vi "运维调试_总磷总氮.vi"() -> ()   [LabVIEW 2016, in "斯坦道总磷总氮.lvlib"]
uses:
  <vilib>/Utility/miscctls.llb/LVPointTypeDef.ctl
  <vilib>/Utility/config.llb/NI_LVConfig.lvlib
  <vilib>/ptbypt/NI_PtbyPt.lvlib
panel:
  in  "模块启用":bool
  in  "串口设置":bool
  in  "备用系数一键写入":bool
  in  "公式一键写入":bool
  in  "流程路径":path=path "C:/Users/std/Documents/斯坦道流程文件/流程.xml"
  in  "曲线模型":cluster{"X^2":dbl, "X":dbl, "B":dbl}(xcontrol)
  out "字符串 2":string
  in  "质控参数设置":bool
  in  "总氮自动测试量程配置":T1
  in  "总磷自动测试量程配置":T1
  out "温度2":sgl
  out "温度1":sgl
  out "ADC":sgl
  out "总氮稀释倍数":dbl
  out "固件版本号":string
  in  "数组":string[](array[string])
  in  "备用系数写入":bool
  in  "备用系数读取":bool
  in  "备用系数":T2
  in  "量程切换阈值写入":bool
  in  "量程切换阈值读取":bool
  in  "量程切换阈值":cluster{"阈值":dbl, "标液浓度":dbl}
  in  "参数下拉列表":enum16{"总磷", "总氮"}(ring)
  in  "量程下拉列表":enum16{"低量程", "高量程"}(ring)
  in  "测量模式下拉列表":enum16{"水样测量", "零点核查", "跨度核查", "标样核查", "加标回收"}(ring)
  in  "公式":cluster{"X^2":dbl, "X":dbl, "b":dbl}
  in  "写公式":bool
  in  "读公式":bool
  in  "返回":bool
  in  "设置":bool
  out "序列号":string="序列号"
  out "总氮测量数据":T3(xcontrol)
  out "总磷测量数据":T3(xcontrol)
  out "集成报警信息":string
  out "定时启动":bool
  out "总磷总氮运行状态":T4(xcontrol)
  in  "停止":bool
  in  "手动启动":bool
  in  "单步测试":bool
  in  "总磷氨氮调试":u16[](xcontrol)
  out "F3":sgl format="%#.6f"
  out "F2":sgl format="%#.6f"
  out "F1":sgl format="%#.6f"
  out "F0":sgl format="%#.6f"
  out "多列列表框":i32(listbox)
  # "参数设置"
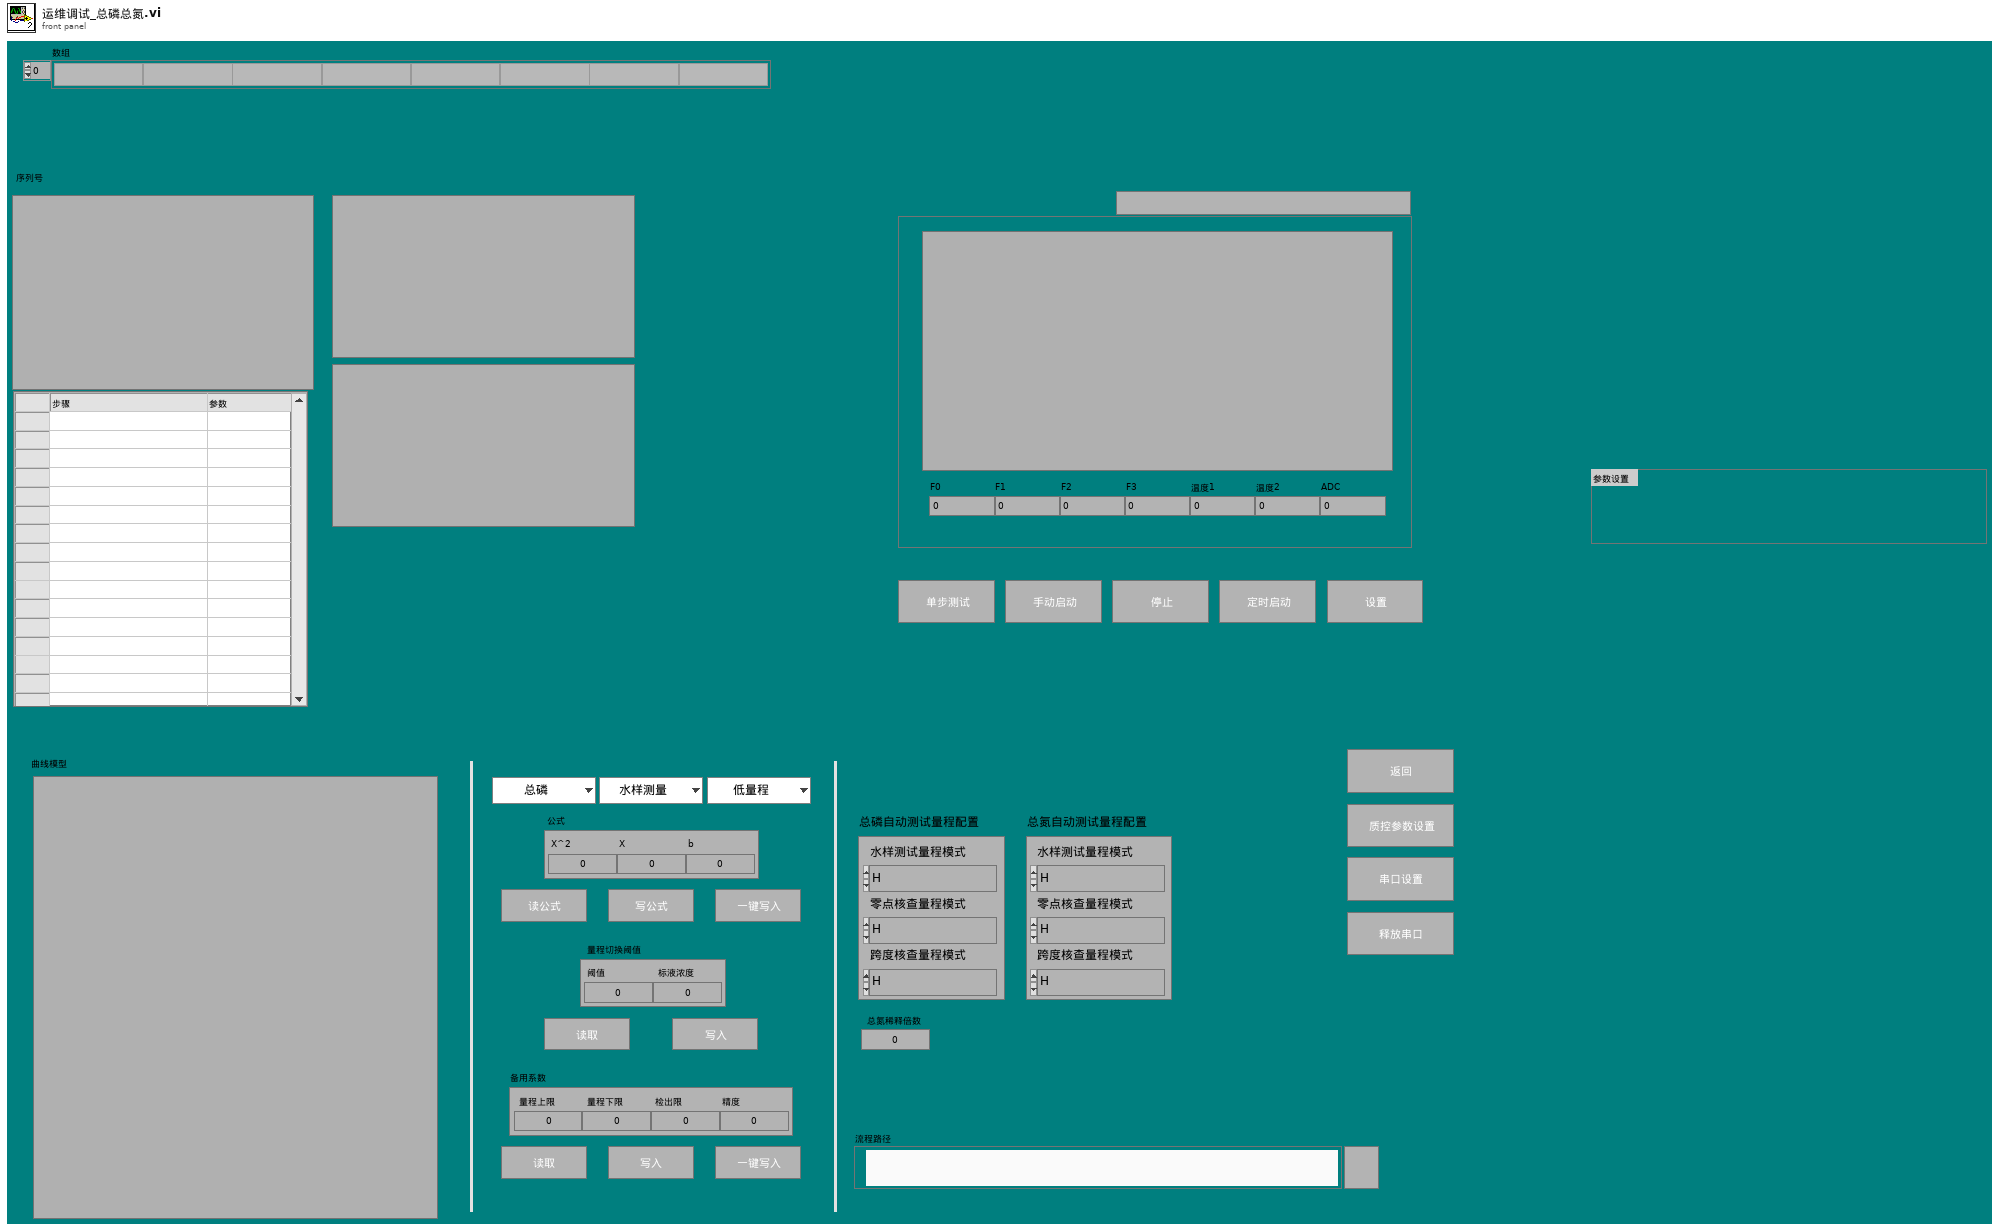
[diagram p1: front panel]
types:
  T1 = cluster{"水样测试量程模式":enum16{"H", "L", "AUTO"}, "空白核查量程模式":enum16{"H", "L", "AUTO"}, "跨度核查量程模式":enum16{"H", "L", "AUTO"}}
  T2 = cluster{"量程上限":dbl, "量程下限":dbl, "检出限":dbl, "精度":dbl}
  T3 = cluster{"flowid":u16, "测量精度":u16, "测量数据区":cluster{"因子编码":u32, "单位":u16, "标样参考值":sgl, "水样数据时间":timestamp, "水样实测值":sgl, "水样数据标识":string, "标样数据时间":timestamp, "标样实测值":sgl, "标样数据标识":string, "空白数据时间":timestamp, "空白实测值":sgl, "空白数据标识":string, "零点核查数据时间":timestamp, "零点核查实测值":sgl, "零点核查数据标识":string, "跨度核查数据时间":timestamp, "跨度核查实测值":sgl, "跨度核查数据标识":string, "加标回收数据时间":timestamp, "加标回收实测值":sgl, "加标回收数据标识":string, "平行样数据时间":timestamp, "平行样实测值":sgl, "平行样数据标识":string, "F0":sgl, "F1":sgl, "F2":sgl, "F3":sgl, "F4":sgl, "F5":sgl, "F6":sgl, "F7":sgl, "温度":sgl, "湿度":sgl, "X值":sgl}}
  T4 = cluster{"系统时间":timestamp, "工作状态":enum16{"空闲", "水样测试", "标样核查", "零点核查", "跨度核查", "空白测试", "平行样测试", "加标回收", "空白校准", "标样校准", "初始化（清洗）"}, "测量模式":enum16{"待机", "连续模式", "周期模式", "定点模式", "受控模式", "手动模式"}, "告警代码":enum16{"无告警", "缺试剂告警", "缺水样告警", "缺蒸馏水告警", "缺标液告警", "仪表漏液告警", "标定异常告警", "超量程告警", "加热异常", "低试剂预警", "超上限告警", "超下限告警", "仪表内部其他异常", "滴定异常告警", "电极异常告警", "量程切换告警", "参数设置告警", "PH电极电位异常", "电导率电极异常", "浊度光度异常", "溶解氧电极异常", "溶解氧光强异常", "温度异常告警", "PH异常告警", "溶解氧异常告警", "电导率异常告警", "浊度异常告警", "叶绿素异常告警", "藻密度异常告警", "蓝绿藻异常告警", "ORP异常告警", "氨氮异常告警", "清洁刷异常告警", "SD卡异常告警", "蓝牙异常告警", "Wifi异常告警", "流程异常告警"}, "故障代码":enum16{"无故障", "电机故障", "温度故障", "通讯故障", "滴定故障"}, "日志代码":u16, "软件版本":u16, "F0":sgl, "F1":sgl, "F2":sgl, "F3":sgl, "T":sgl, "H":sgl, "id":u16, "flowid":u16, "量程":u16, "总磷控温温度1":sgl, "营养盐控温温度2":sgl, "ADC":sgl}
  T5 = enum16{"启动测量", "标样核查", "零点核查", "跨度核查", "空白测试", "平行样测试", "加标回收", "空白校准", "标样校准", "初始化（清洗）", "停止测试", "仪器重启", "校时", "模式设置", "测量间隔设置"}
  T6 = cluster{"仪器测试类型":enum16{"启动测量", "标样核查", "零点核查", "跨度核查", "空白测试", "平行样测试", "加标回收", "空白校准", "标样校准", "初始化（清洗）", "停止测试", "仪器重启", "校时", "模式设置", "测量间隔设置"}, "周期设置类型":enum16{"定点启动", "间隔启动"}, "定时功能启用":bool, "定时间隔":dbl, "24H周期设置":bool[], "零点核查时间":u16, "跨度核查时间":u16, "质控频次":enum16{"关闭", "每天", "星期一", "星期二", "星期三", "星期四", "星期五", "星期六", "星期日"}}
  T7 = enum16{"关闭", "每天", "星期一", "星期二", "星期三", "星期四", "星期五", "星期六", "星期日"}
  T8 = enum32{"Bad", "Idle", "Run top level", "Running"}
  T9 = typedef "LVDateTimeRec.ctl" = cluster{"秒数的小数部分":dbl, "秒":i32, "分":i32, "时":i32, "日":i32, "月":i32, "年":i32, "天数（周）":i32, "天数（年）":i32, "DST":i32}
  T10 = typedef "LVPointTypeDef.ctl" = cluster{"Horizontal":i16, "Vertical":i16}
  T11 = cluster{"因子编码":u32, "单位":u16, "标样参考值":sgl, "水样数据时间":timestamp, "水样实测值":sgl, "水样数据标识":string, "标样数据时间":timestamp, "标样实测值":sgl, "标样数据标识":string, "空白数据时间":timestamp, "空白实测值":sgl, "空白数据标识":string, "零点核查数据时间":timestamp, "零点核查实测值":sgl, "零点核查数据标识":string, "跨度核查数据时间":timestamp, "跨度核查实测值":sgl, "跨度核查数据标识":string, "加标回收数据时间":timestamp, "加标回收实测值":sgl, "加标回收数据标识":string, "平行样数据时间":timestamp, "平行样实测值":sgl, "平行样数据标识":string, "F0":sgl, "F1":sgl, "F2":sgl, "F3":sgl, "F4":sgl, "F5":sgl, "F6":sgl, "F7":sgl, "温度":sgl, "湿度":sgl, "X值":sgl}
  T12 = enum16{"空闲", "水样测试", "标样核查", "零点核查", "跨度核查", "空白测试", "平行样测试", "加标回收", "空白校准", "标样校准", "初始化（清洗）"}
  T13 = typedef "NI_LVConfig.lvlib/Config Data RefNum.ctl" = refnum<k1>
  T14 = cluster{"启动模式":enum16{"跨度核查", "水样测量", "空白核查", "标样核查", "加标回收"}, "启动参数":u16, "量程":enum16{"低量程", "高量程"}}
  T15 = cluster{"时间标识":timestamp, "设备":string, "日志信息":string, "流程参数":string}
  T16 = cluster{"时间标识":timestamp, "设备":string, "日志信息":string}
  T17 = enum16{"无告警", "缺试剂告警", "缺水样告警", "缺蒸馏水告警", "缺标液告警", "仪表漏液告警", "标定异常告警", "超量程告警", "加热异常", "低试剂预警", "超上限告警", "超下限告警", "仪表内部其他异常", "滴定异常告警", "电极异常告警", "量程切换告警", "参数设置告警", "PH电极电位异常", "电导率电极异常", "浊度光度异常", "溶解氧电极异常", "溶解氧光强异常", "温度异常告警", "PH异常告警", "溶解氧异常告警", "电导率异常告警", "浊度异常告警", "叶绿素异常告警", "藻密度异常告警", "蓝绿藻异常告警", "ORP异常告警", "氨氮异常告警", "清洁刷异常告警", "SD卡异常告警", "蓝牙异常告警", "Wifi异常告警", "流程异常告警"}
  T18 = typedef "LVRowAndColumnUnsignedTypeDef.ctl" = cluster{"Row":u32, "Column":u32}
  T19 = cluster{"参数下拉列表":enum16{"总磷", "总氮"}, "测量模式下拉列表":enum16{"水样测量", "零点核查", "跨度核查", "标样核查", "加标回收"}, "量程下拉列表":enum16{"低量程", "高量程"}}
  T20 = cluster{"站号":u16, "量程切换":enum32{"H", "L", "AUTO"}, "控制命令":enum16{"启动测量", "标样核查", "零点核查", "跨度核查", "空白测试", "平行样测试", "加标回收", "空白校准", "标样校准", "初始化（清洗）", "停止测试", "仪器重启", "校时", "模式设置", "测量间隔设置"}, "模式设置":enum16{"待机", "连续模式", "周期模式", "定点模式", "受控模式", "手动模式"}, "测量间隔":u16}
  T21 = cluster{"总磷跨度值":dbl, "总磷零点标准液浓度":dbl, "总磷跨度标准液浓度":dbl, "总磷标准液标准浓度":dbl, "总氮跨度值":dbl, "总氮零点标准液浓度":dbl, "总氮跨度标准液浓度":dbl, "总氮标准液标准浓度":dbl}
  T22 = cluster{"确定":bool, "总磷跨度值":dbl, "总磷零点标准液浓度":dbl, "总磷跨度标准液浓度":dbl, "总磷标准液标准浓度":dbl, "总氮跨度值":dbl, "总氮零点标准液浓度":dbl, "总氮跨度标准液浓度":dbl, "总氮标准液标准浓度":dbl}
  T23 = cluster{"控制命令":enum16{"启动测量", "标样核查", "零点核查", "跨度核查", "空白测试", "平行样测试", "加标回收", "空白校准", "标样校准", "初始化（清洗）", "停止测试", "仪器重启", "校时", "模式设置", "测量间隔设置"}, "周期设置类型":enum16{"定点启动", "间隔启动"}, "定时功能启用":bool, "定时间隔":dbl, "24H周期设置":bool[], "空白核查时间":u16, "跨度核查时间":u16, "质控频次":enum16{"关闭", "每天", "星期一", "星期二", "星期三", "星期四", "星期五", "星期六", "星期日"}}
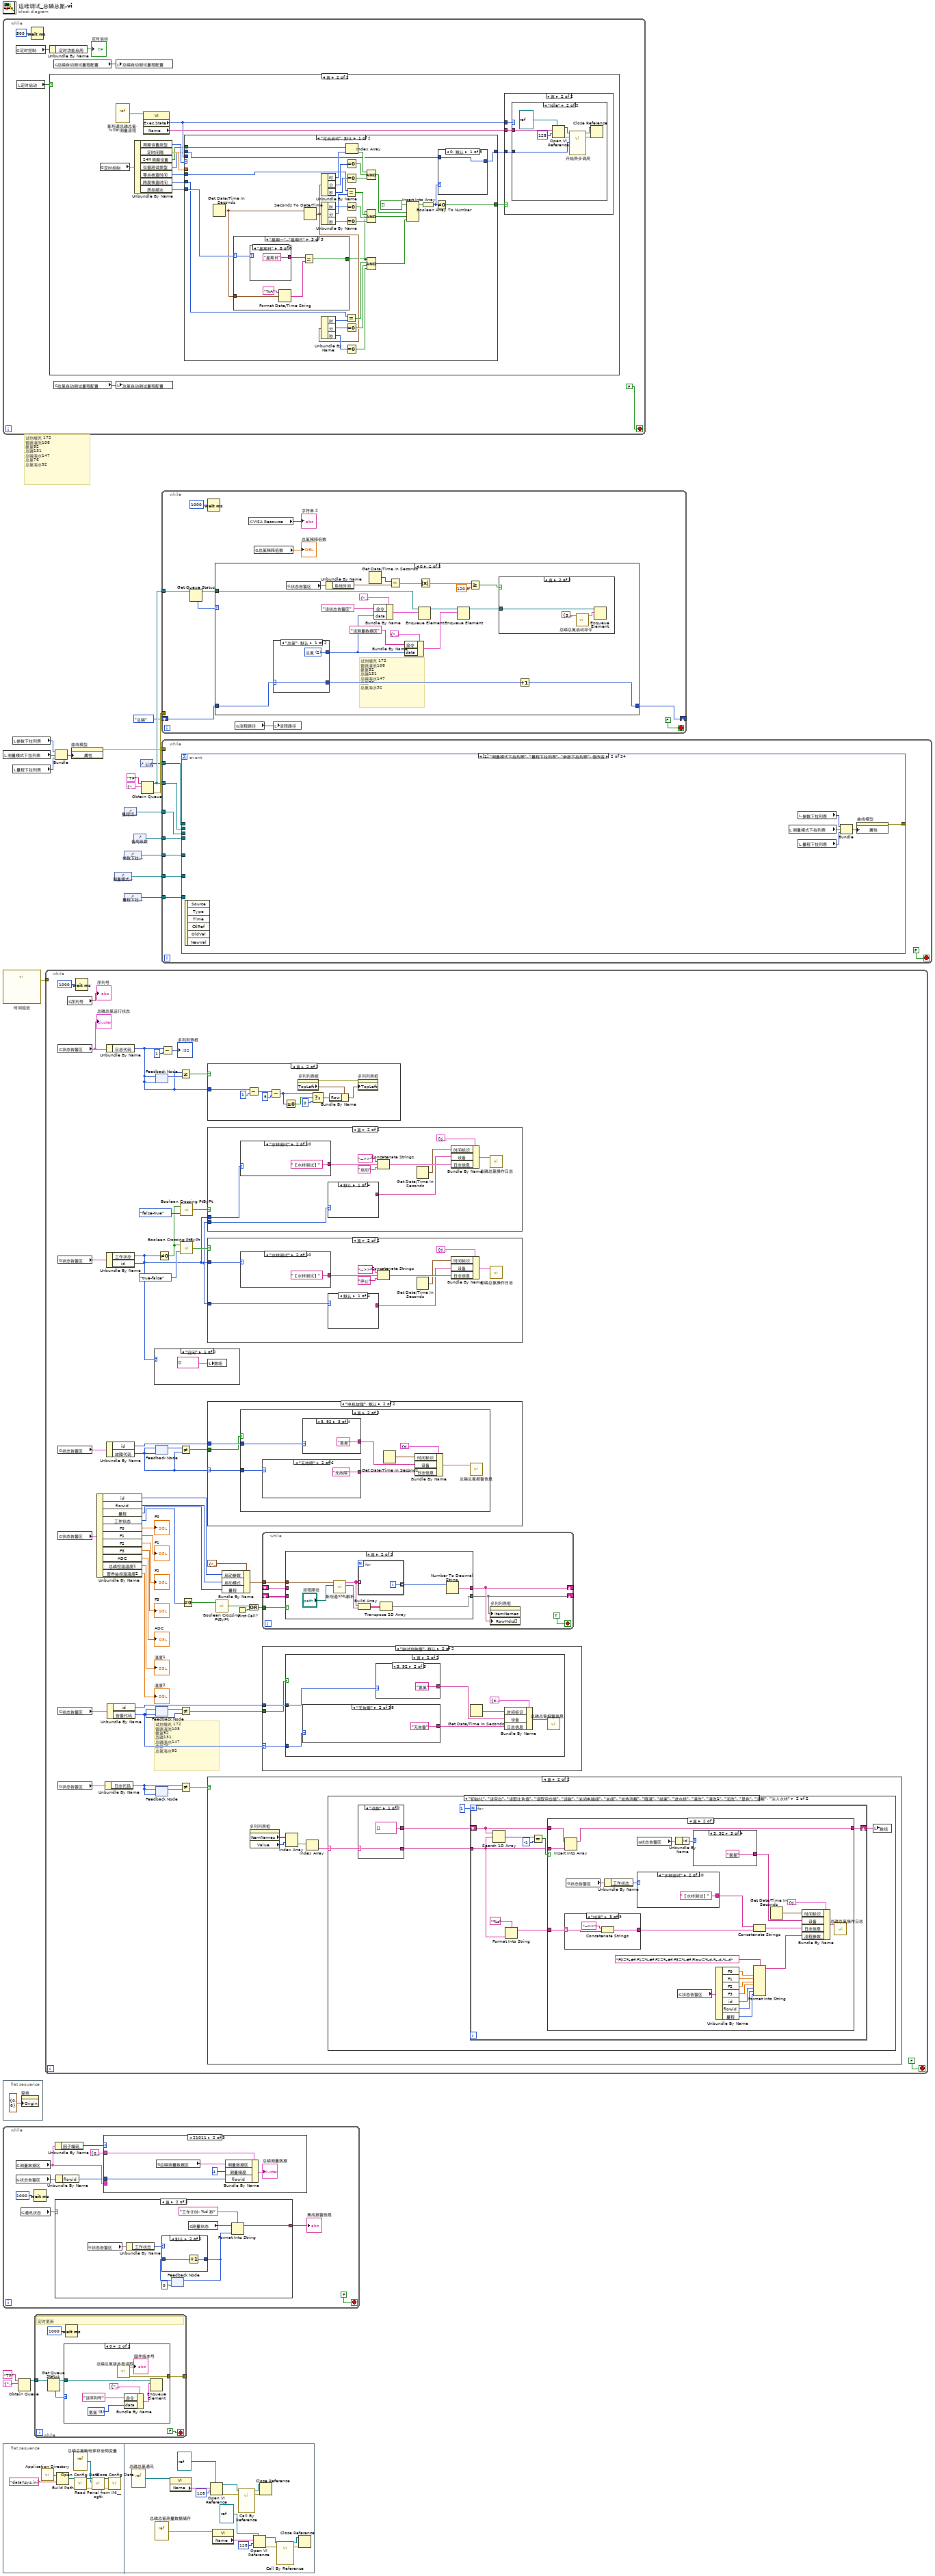
[diagram p0: block diagram]
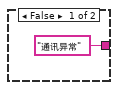
[diagram p3: hidden frame]
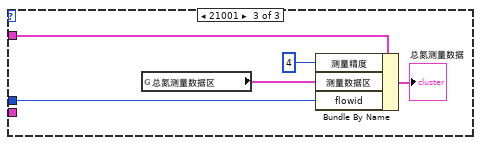
[diagram p6: hidden frame]
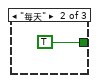
[diagram p9: hidden frame]
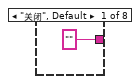
[diagram p10: hidden frame]
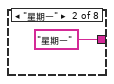
[diagram p11: hidden frame]
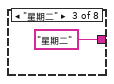
[diagram p12: hidden frame]
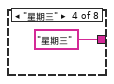
[diagram p13: hidden frame]
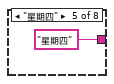
[diagram p14: hidden frame]
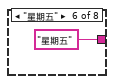
[diagram p15: hidden frame]
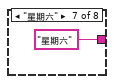
[diagram p16: hidden frame]
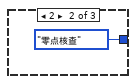
[diagram p17: hidden frame]
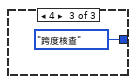
[diagram p18: hidden frame]
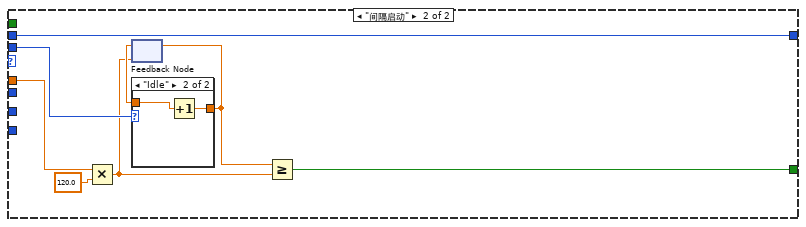
[diagram p19: hidden frame]
diagram:
  # "试剂填充 172 \n管路清洗108\n氨氮92\n总磷131\n总磷海水147\n总氮76\n总氮海水92"
  n1 = while {
    stop <- FALSE stop-if-true
    n2 = global read "总磷总氮断电保存全局变量.vi" "定时控制"() -> (w22:T6)
    n3 = local read "定时启动"() -> (w25:bool)
    n4 = Wait (ms)(milliseconds to wait=u32 500 ("等待时间（毫秒）")) -> ()  [unwired: 1 out]
    n5 = Unbundle By Name(w22) -> ("定时功能启用"=→"定时启动":bool)
    n6 = case shown="真" w25 {
      frame False {
      }
      frame True {
        n7 = global read "总磷总氮断电保存全局变量.vi" "定时控制"() -> (w40:T6)
        n8 = vi-ref "斯坦道总磷总氮.lvlib:测量流程.vi"() -> (w39:refnum<vi>)
        n9 = Unbundle By Name(w40) -> ("周期设置类型"=w37:enum16{"定点启动", "间隔启动"}, "定时间隔"=w35:dbl, "24H周期设置"=w34:bool[], "仪器测试类型"=w33:T5, "零点核查时间"=w32:u16, "跨度核查时间"=w31:u16, "质控频次"=w30:T7)
        n10 = property class="VI"(reference=w39) -> ("Exec.State"=w36:T8, "Name"=w38:string)  [unwired: 1 in, 2 out]
        n11 = case shown="\"定点启动\", 默认" w37 {
          tunnel: w35 -> [_ w97]
          tunnel: w34 -> [w65 _]
          tunnel: w36 -> [_ w100]
          tunnel: [w43 w95] -> w28
          tunnel: w33 -> [w41 w93]
          tunnel: [w69 w93] -> w29
          tunnel: w30 -> [w68 _]
          tunnel: w32 -> [w61 _]
          tunnel: w31 -> [w50 _]
          frame "定点启动", Default {
            n12 = Get Date/Time In Seconds() -> (seconds since 1Jan1904=w67:timestamp)
            n13 = case shown="\"星期一\"..\"星期日\"" w68 {
              selector: w68 -> [_ _ w79]
              tunnel: w67 -> [_ _ w80]
              tunnel: [_ TRUE w76] -> w49
              frame "关闭", Default {
              }
              frame "每天" {
              }
              frame "星期一".."星期日" {
                n14 = case shown="\"星期日\"" w79 {
                  tunnel: ["" ("时间格式字符串(%c)") "星期一" ("时间格式字符串(%c)") "星期二" ("时间格式字符串(%c)") "星期三" ("时间格式字符串(%c)") "星期四" ("时间格式字符串(%c)") "星期五" ("时间格式字符串(%c)") "星期六" ("时间格式字符串(%c)") "星期日" ("时间格式字符串(%c)")] -> w78
                  frame "关闭", Default {
                  }
                  frame "星期一" {
                  }
                  frame "星期二" {
                  }
                  frame "星期三" {
                  }
                  frame "星期四" {
                  }
                  frame "星期五" {
                  }
                  frame "星期六" {
                  }
                  frame "星期日" {
                  }
                }
                n15 = Format Date/Time String(time format string (%c)="%A" ("时间格式字符串(%c)"), seconds (now)=w80) -> (date/time string=w77:string)  [unwired: 1 in]
                n16 = Equal?(x=w78, y=w77) -> (x = y?=w76:bool)
              }
            }
            n17 = Seconds To Date/Time(time stamp (now)=w67) -> (date time rec=w51:T9)  [unwired: 1 in]
            n18 = Unbundle By Name(w51) -> ("时"=w74:i32, "分"=w72:i32, "秒"=w73:i32)
            n19 = Unbundle By Name(w51) -> ("时"=w62:i32, "分"=w64:i32, "秒"=w63:i32)
            n20 = Unbundle By Name(w51) -> ("时"=w54:i32, "分"=w52:i32, "秒"=w53:i32)
            n21 = Equal?(x=w61, y=w62) -> (x = y?=w60:bool)
            n22 = Equal?(x=w50, y=w54) -> (x = y?=w55:bool)
            n23 = Equal To 0?(x=w72) -> (x = 0?=w71:bool)
            n24 = Equal To 0?(x=w73) -> (x = 0?=w70:bool)
            n25 = Equal To 0?(x=w64) -> (x = 0?=w59:bool)
            n26 = Equal To 0?(x=w63) -> (x = 0?=w58:bool)
            n27 = Equal To 0?(x=w52) -> (x = 0?=w56:bool)
            n28 = Equal To 0?(x=w53) -> (x = 0?=w57:bool)
            n29 = Index Array(array=w65, index=w74) -> (element=w66:bool)
            n30 = Compound Arithmetic op=AND ("复合运算")(w66, w71, w70) -> (w47:bool)
            n31 = Compound Arithmetic op=AND ("复合运算")(w49, w60, w59, w58) -> (w46:bool)
            n32 = Compound Arithmetic op=AND ("复合运算")(w49, w55, w56, w57) -> (w45:bool)
            n33 = Insert Into Array(array=bool[] [], new element #1=w47, new element #2=w46, new element #3=w45) -> (w44:bool[])  [unwired: 1 in]
            n34 = Boolean Array To Number(Boolean array=w44) -> (number=w42:u32)
            n35 = Not Equal To 0?(x=w42) -> (x != 0?=w43:bool)
            n36 = case shown="0, 默认" w42 {
              tunnel: [w90 T5."零点核查" ("控制命令") T5."跨度核查" ("控制命令")] -> w69
              tunnel: w41 -> [w90 _ _]
              frame 0, Default {
              }
              frame 2 {
              }
              frame 4 {
              }
            }
          }
          frame "间隔启动" {
            n37 = Multiply(x=w97, y=120.0) -> (x*y=w94:dbl)
            n38 = feedback #1(w94) -> (w99:dbl)
            n39 = case shown="\"Idle\"" w100 {
              tunnel: w99 -> [_ w102]
              tunnel: [_ w101] -> w98
              frame "Bad", Default {
              }
              frame "Idle" {
                n40 = Increment(x=w102) -> (x+1=w101:dbl)
              }
            }
            n41 = feedback-in #1(w98) -> ()
            n42 = Greater Or Equal?(x=w98, y=w94) -> (x >= y?=w95:bool)
          }
        }
        n43 = case shown="真" w28 {
          tunnel: w38 -> [_ w105]
          tunnel: w29 -> [_ w104]
          tunnel: w36 -> [_ w103]
          frame False {
          }
          frame True {
            n44 = case shown="\"Idle\"" w103 {
              tunnel: w105 -> [_ w109]
              tunnel: w104 -> [_ w106]
              frame "Bad", Default {
              }
              frame "Idle" {
                n45 = Open VI Reference(type specifier VI Refnum (for type only)=refnum<vi> refnum, vi path=w109, options=128 ("选项")) -> (vi reference=w110:refnum<vi>, error out=w111:errorcluster)  [unwired: 3 in]
                n46 = call-by-ref "开始异步调用"(reference=w110, error in=w111, "控制命令"=w106) -> (reference out=w112:refnum<vi>, error out=w113:errorcluster)  [unwired: 11 in]
                n47 = Close Reference(reference=w112, error in (no error)=w113) -> ()  [unwired: 1 out]
              }
            }
          }
        }
      }
    }
    n48 = global read "总磷总氮断电保存全局变量.vi" "总磷自动测试量程配置"() -> (w23:T1)
    n49 = global read "总磷总氮断电保存全局变量.vi" "总氮自动测试量程配置"() -> (w24:T1)
    n50 = local write "总磷自动测试量程配置"(w23) -> ()
    n51 = local write "总氮自动测试量程配置"(w24) -> ()
  }
  n52 = local read "测量模式下拉列表"() -> (w3:enum16{"水样测量", "零点核查", "跨度核查", "标样核查", "加标回收"})
  n53 = call "时间延迟"() -> ("error out"=w9:errorcluster)  [unwired: 11 in]
  n54 = flat-sequence {
    frame #0 {
      n55 = property on="窗格" class="Pane"("Origin"=T10 {"Horizontal"=0, "Vertical"=0} ("原点")) -> ()  [unwired: 2 in, 2 out]
    }
  }
  n56 = while {
    stop <- FALSE stop-if-true
    n57 = global read "VAR总磷总氮全局变量.vi" "测量数据区"() -> (w121:T11)
    n58 = global read "VAR总磷总氮全局变量.vi" "状态告警区"() -> (w117:T4)
    n59 = global read "VAR总磷总氮全局变量.vi" "通讯状态"() -> (w119:bool)
    n60 = Wait (ms)(milliseconds to wait=u32 1000 ("等待时间（毫秒）")) -> ()  [unwired: 1 out]
    n61 = Unbundle By Name(w121) -> ("因子编码"=w120:u32)
    n62 = case shown="真" w119 {
      tunnel: ["通讯异常" ("集成报警信息") w126] -> w118
      frame False {
      }
      frame True {
        n63 = global read "VAR总磷总氮全局变量.vi" "状态告警区"() -> (w132:T4)
        n64 = Unbundle By Name(w132) -> ("工作状态"=w131:T12)
        n65 = feedback #2(0) -> (w129:i32)
        n66 = case shown="默认" w131 {
          tunnel: w129 -> [_ w134]
          tunnel: [_ w133] -> w127
          frame "空闲" {
          }
          frame Default {
            n67 = Increment(x=w134) -> (x+1=w133:i32)
          }
        }
        n68 = feedback-in #2(w127) -> ()
        n69 = global read "VAR总磷总氮全局变量.vi" "测量状态"() -> (w125:string)
        n70 = Format Into String(format string="工作计时: %d 秒" ("格式字符串"), initial string=w125, w127) -> (resulting string=w126:string)  [unwired: 1 in, 1 out]
      }
    }
    "集成报警信息" <- w118
    n71 = Unbundle By Name(w117) -> ("flowid"=w116:u16)
    n72 = case shown="21011" w120 {
      tunnel: w121 -> [_ _ _]
      tunnel: w116 -> [_ w137 w143]
      tunnel: T3 {"flowid"=0, "测量精度"=0, "测量数据区"={"因子编码"=0, "单位"=0, "标样参考值"=0.0, "水样数据时间"=timestamp(0 s since 1904-01-01), "水样实测值"=0.0, "水样数据标识"="", "标样数据时间"=timestamp(0 s since 1904-01-01), "标样实测值"=0.0, "标样数据标识"="", "空白数据时间"=timestamp(0 s since 1904-01-01), "空白实测值"=0.0, "空白数据标识"="", "零点核查数据时间"=timestamp(0 s since 1904-01-01), "零点核查实测值"=0.0, "零点核查数据标识"="", "跨度核查数据时间"=timestamp(0 s since 1904-01-01), "跨度核查实测值"=0.0, "跨度核查数据标识"="", "加标回收数据时间"=timestamp(0 s since 1904-01-01), "加标回收实测值"=0.0, "加标回收数据标识"="", "平行样数据时间"=timestamp(0 s since 1904-01-01), "平行样实测值"=0.0, "平行样数据标识"="", "F0"=0.0, "F1"=0.0, "F2"=0.0, "F3"=0.0, "F4"=0.0, "F5"=0.0, "F6"=0.0, "F7"=0.0, "温度"=0.0, "湿度"=0.0, "X值"=0.0}} ("总氮测量数据") -> [_ w136 w142]
      frame Default {
      }
      frame 21011 {
        n73 = global read "VAR总磷总氮全局变量.vi" "总磷测量数据区"() -> (w135:T11)
        n74 = Bundle By Name(cluster=w136, "测量数据区"=w135, "测量精度"=u16 4, "flowid"=w137) -> (→"总磷测量数据":T3)
      }
      frame 21001 {
        n75 = global read "VAR总磷总氮全局变量.vi" "总氮测量数据区"() -> (w140:T11)
        n76 = Bundle By Name(cluster=w142, "测量精度"=u16 4, "测量数据区"=w140, "flowid"=w143) -> (→"总氮测量数据":T3)
      }
    }
  }
  n77 = flat-sequence {
    frame #0 {
      n78 = call <vilib>:"Application Directory.vi"() -> ("Application Directory"=w152:path)
      n79 = Build Path(base path=w152, name or relative path="data\\sys.ini" ("名称或相对路径")) -> (appended path=w150:path)
      n80 = vi-ref "总磷总氮断电保存全局变量.vi"() -> (w148:refnum<vi>)
      n81 = call <vilib>:"Open Config Data.vi"("configuration file path"=w150) -> ("error out"=w146:errorcluster, "refnum"=w149:T13)  [unwired: 8 in, 1 out]
      n82 = call <userlib>:"Read Panel from INI__ogtk.vi"("error in (no error)"=w146, "VI ref"=w148, "refnum"=w149) -> ("error out"=w145:errorcluster, "refnum out"=w147:T13)  [unwired: 7 in]
      n83 = call <vilib>:"Close Config Data.vi"("error in (no error)"=w145, "refnum"=w147) -> ()  [unwired: 8 in, 2 out]
    }
    frame #1 {
      n84 = vi-ref "总磷总氮通讯.vi"() -> (w168:refnum<vi>)
      n85 = vi-ref "总磷总氮测量数据储存.vi"() -> (w160:refnum<vi>)
      n86 = property class="VI"(reference=w168) -> ("Name"=w167:string)  [unwired: 1 in, 2 out]
      n87 = Open VI Reference(type specifier VI Refnum (for type only)=refnum<vi> refnum, vi path=w167, options=128 ("选项")) -> (vi reference=w165:refnum<vi>, error out=w163:errorcluster)  [unwired: 3 in]
      n88 = property class="VI"(reference=w160) -> ("Name"=w153:string)  [unwired: 1 in, 2 out]
      n89 = call-by-ref "?"(reference=w165, error in=w163) -> (reference out=w161:refnum<vi>, error out=w162:errorcluster)  [unwired: 12 in]
      n90 = Open VI Reference(type specifier VI Refnum (for type only)=refnum<vi> refnum, vi path=w153, options=128 ("选项")) -> (vi reference=w155:refnum<vi>, error out=w157:errorcluster)  [unwired: 3 in]
      n91 = Close Reference(reference=w161, error in (no error)=w162) -> ()  [unwired: 1 out]
      n92 = call-by-ref "?"(reference=w155, error in=w157) -> (reference out=w159:refnum<vi>, error out=w158:errorcluster)  [unwired: 12 in]
      n93 = Close Reference(reference=w159, error in (no error)=w158) -> ()  [unwired: 1 out]
    }
  }
  n94 = local read "参数下拉列表"() -> (w2:enum16{"总磷", "总氮"})
  n95 = local read "量程下拉列表"() -> (w1:enum16{"低量程", "高量程"})
  n96 = Obtain Queue(name (unnamed)="TP" ("名称（未命名）"), element data type=cluster{"命令":string, "data":variant} {"命令"="", "data"=variant}) -> (queue out=w6:refnum<queue>)  [unwired: 3 in, 2 out]
  n97 = while {
    tunnel: w6 -> [w173]
    tunnel: [w171] -> _
    stop <- FALSE stop-if-true
    # "定时更新"
    n98 = Get Queue Status(queue=w173) -> (queue out=w170:refnum<queue>, # elements in queue=w169:i32)  [unwired: 2 in, 6 out]
    n99 = case shown="0" w169 {
      tunnel: w170 -> [_ w178]
      tunnel: [_ w175] -> w171
      frame Default {
      }
      frame 0 {
        w179 = u16 3 items=["总磷"=1, "氨氮"=3] ("站号")
        n100 = call "总磷总氮版本号读取.vi"() -> ("error out"=w175:errorcluster, "固件版本号"=→"固件版本号":string)  [unwired: 10 in]
        n101 = Bundle By Name(cluster=cluster{"命令":string, "data":variant} {"命令"="", "data"=variant} ("元素"), "命令"="读序列号", "data"=w179) -> (w177:cluster{"命令":string, "data":variant})
        n102 = Enqueue Element(queue=w178, element=w177) -> ()  [unwired: 2 in, 3 out]
      }
    }
    n103 = Wait (ms)(milliseconds to wait=u32 1000 ("等待时间（毫秒）")) -> ()  [unwired: 1 out]
  }
  n104 = while {
    tunnel: w9 -> [_]
    stop <- FALSE stop-if-true
    # "试剂填充 172 \n管路清洗108\n氨氮92\n总磷131\n总磷海水147\n总氮76\n总氮海水92"
    n105 = global read "VAR总磷总氮全局变量.vi" "状态告警区"() -> (w215:T4)
    "总磷总氮运行状态" <- w215
    n106 = global read "VAR总磷总氮全局变量.vi" "状态告警区"() -> (w202:T4)
    n107 = global read "VAR总磷总氮全局变量.vi" "状态告警区"() -> (w207:T4)
    n108 = global read "VAR总磷总氮全局变量.vi" "状态告警区"() -> (w223:T4)
    n109 = global read "VAR总磷总氮全局变量.vi" "状态告警区"() -> (w212:T4)
    n110 = global read "VAR总磷总氮全局变量.vi" "状态告警区"() -> (w200:T4)
    n111 = global read "VAR总磷总氮全局变量.vi" "序列号"() -> (→"序列号":string)
    n112 = Wait (ms)(milliseconds to wait=u32 1000 ("等待时间（毫秒）")) -> ()  [unwired: 1 out]
    n113 = Unbundle By Name(w223) -> ("id"=w220:u16, "flowid"=w222:u16, "量程"=w221:u16, "工作状态"=w190:T12, "F0"=→"F0":sgl, "F1"=→"F1":sgl, "F2"=→"F2":sgl, "F3"=→"F3":sgl, "ADC"=→"ADC":sgl, "总磷控温温度1"=→"温度1":sgl, "营养盐控温温度2"=→"温度2":sgl)
    n114 = Unbundle By Name(w200) -> ("日志代码"=w199:u16)
    n115 = Unbundle By Name(w215) -> ("日志代码"=w196:u16)
    n116 = Unbundle By Name(w202) -> ("工作状态"=w183:T12, "id"=w182:u16)
    n117 = Unbundle By Name(w207) -> ("id"=w206:u16, "故障代码"=w203:enum16{"无故障", "电机故障", "温度故障", "通讯故障", "滴定故障"})
    n118 = Unbundle By Name(w212) -> ("id"=w211:u16, "告警代码"=w208:T17)
    n119 = case shown="\"空闲\"" w183 {
      frame "空闲" {
        n120 = local write "数组"(string[] [] ("数组")) -> ()
      }
      frame "水样测试", Default {
      }
    }
    n121 = feedback-in #3(w196) -> ()
    n122 = feedback #3(w196) -> (w228:u16)
    n123 = feedback #4(w203) -> (w204:enum16{"无故障", "电机故障", "温度故障", "通讯故障", "滴定故障"})
    n124 = feedback-in #4(w203) -> ()
    n125 = feedback #5(w208) -> (w209:T17)
    n126 = feedback-in #5(w208) -> ()
    n127 = feedback #6(w199) -> (w201:u16)
    n128 = feedback-in #6(w199) -> ()
    n129 = Not Equal To 0?(x=w183) -> (x != 0?=w185:bool)
    n130 = Subtract(x=w196, y=1) -> (x-y=→"多列列表框":i32)
    n131 = Not Equal?(x=w196, y=w228) -> (x != y?=w227:bool)
    n132 = Not Equal?(x=w204, y=w203) -> (x != y?=w205:bool)
    n133 = Not Equal?(x=w209, y=w208) -> (x != y?=w210:bool)
    n134 = Not Equal?(x=w199, y=w201) -> (x != y?=w198:bool)
    n135 = call <vilib>:"Boolean Crossing PtByPt.vi"("direction"=enum16{"either", "false-true", "true-false"}."false-true", "input"=w185) -> ("crossing"=w187:bool)  [unwired: 1 in]
    n136 = call <vilib>:"Boolean Crossing PtByPt.vi"("direction"=enum16{"either", "false-true", "true-false"}."true-false", "input"=w185) -> ("crossing"=w184:bool)  [unwired: 1 in]
    n137 = Not Equal To 0?(x=w190) -> (x != 0?=w225:bool)
    n138 = case shown="真" w227 {
      tunnel: w196 -> [_ w438]
      frame False {
      }
      frame True {
        n139 = Subtract(x=w438, y=1) -> (x-y=w436:i32)
        n140 = Subtract(x=w436, y=5) -> (x-y=w440:i32)
        n141 = Greater Or Equal To 0?(x=w440) -> (x >= 0?=w439:bool)
        n142 = property on="多列列表框" class="MCListbox (严格)"() -> (error out=w444:errorcluster, "TopLeft"=w445:T18)  [unwired: 2 in, 1 out]
        n143 = Select(t=w440, s=w439, f=0) -> (s? t:f=w441:i32)
        n144 = Bundle By Name(cluster=w445, "Row"=w441) -> (w446:T18)
        n145 = property on="多列列表框" class="MCListbox (严格)"(error in=w444, "TopLeft"=w446) -> ()  [unwired: 1 in, 2 out]
      }
    }
    n146 = case shown="真" w187 {
      tunnel: w183 -> [_ w255]
      tunnel: w182 -> [_ w254]
      frame False {
      }
      frame True {
        n147 = case shown="\"水样测试\"" w255 {
          tunnel: [_ "【水样测试】" ("字符串") "【标样核查】" ("字符串") "【零点核查】" ("字符串") "【跨度核查】" ("字符串") "【空白测试】" ("字符串") "【平行样测试】" ("字符串") "【加标回收】" ("字符串") "【空白校准】" ("字符串") "【标样校准】" ("字符串")] -> w262
          frame "空闲", Default {
          }
          frame "水样测试" {
          }
          frame "标样核查" {
          }
          frame "零点核查" {
          }
          frame "跨度核查" {
          }
          frame "空白测试" {
          }
          frame "平行样测试" {
          }
          frame "加标回收" {
          }
          frame "空白校准" {
          }
          frame "标样校准" {
          }
        }
        n148 = case shown="默认" w254 {
          tunnel: [_ "总磷" ("table输入") "氨氮" ("table输入") "总氮" ("table输入")] -> w258
          frame Default {
          }
          frame 1, 131 {
          }
          frame 3, 92 {
          }
          frame 2, 76 {
          }
        }
        n149 = Concatenate Strings("-->>" ("字符串"), w262, "启动" ("字符串")) -> (w261:string)
        n150 = Get Date/Time In Seconds() -> (seconds since 1Jan1904=w259:timestamp)
        n151 = Bundle By Name(cluster=T15 {"时间标识"=timestamp(0 s since 1904-01-01), "设备"="", "日志信息"="", "流程参数"=""} ("data in"), "时间标识"=w259, "设备"=w258, "日志信息"=w261) -> (w253:T15)
        n152 = call "总磷总氮操作日志.vi"("data in"=w253) -> ()  [unwired: 11 in]
      }
    }
    n153 = case shown="真" w184 {
      tunnel: w183 -> [_ w233]
      tunnel: w182 -> [_ w232]
      frame False {
      }
      frame True {
        n154 = case shown="\"水样测试\"" w233 {
          tunnel: [_ "【水样测试】" ("字符串") "【标样核查】" ("字符串") "【零点核查】" ("字符串") "【跨度核查】" ("字符串") "【空白测试】" ("字符串") "【平行样测试】" ("字符串") "【加标回收】" ("字符串") "【空白校准】" ("字符串") "【标样校准】" ("字符串")] -> w240
          frame "空闲", Default {
          }
          frame "水样测试" {
          }
          frame "标样核查" {
          }
          frame "零点核查" {
          }
          frame "跨度核查" {
          }
          frame "空白测试" {
          }
          frame "平行样测试" {
          }
          frame "加标回收" {
          }
          frame "空白校准" {
          }
          frame "标样校准" {
          }
        }
        n155 = case shown="默认" w232 {
          tunnel: [_ "总磷" ("table输入") "氨氮" ("table输入") "总氮" ("table输入")] -> w236
          frame Default {
          }
          frame 1, 131 {
          }
          frame 3, 92 {
          }
          frame 2, 76 {
          }
        }
        n156 = Concatenate Strings("-->>" ("字符串"), w240, "停止" ("字符串")) -> (w239:string)
        n157 = Get Date/Time In Seconds() -> (seconds since 1Jan1904=w237:timestamp)
        n158 = Bundle By Name(cluster=T15 {"时间标识"=timestamp(0 s since 1904-01-01), "设备"="", "日志信息"="", "流程参数"=""} ("data in"), "时间标识"=w237, "设备"=w236, "日志信息"=w239) -> (w231:T15)
        n159 = call "总磷总氮操作日志.vi"("data in"=w231) -> ()  [unwired: 11 in]
      }
    }
    n160 = case shown="\"电机故障\", 默认" w203 {
      selector: w203 -> [_ w343]
      tunnel: w206 -> [_ w344]
      tunnel: w205 -> [_ w342]
      frame "无故障" {
      }
      frame "电机故障", Default {
        n161 = case shown="真" w342 {
          tunnel: w344 -> [_ w351]
          tunnel: w343 -> [_ w346]
          frame False {
          }
          frame True {
            n162 = case shown="\"无故障\"" w346 {
              selector: w346 -> [w353 _ _ _ _ _]
              tunnel: [w352 "无故障" "电机故障" "温度故障" "通讯故障" "滴定故障"] -> w345
              frame Default {
                n163 = Format Into String(format string="%d" ("格式字符串"), initial string="未知" ("工作状态"), w353) -> (resulting string=w352:string)  [unwired: 1 in, 1 out]
              }
              frame "无故障" {
              }
              frame "电机故障" {
              }
              frame "温度故障" {
              }
              frame "通讯故障" {
              }
              frame "滴定故障" {
              }
            }
            n164 = case shown="3, 92" w351 {
              tunnel: [_ "总磷" ("table输入") "氨氮" ("table输入") "总氮" ("table输入")] -> w347
              frame Default {
              }
              frame 1, 131 {
              }
              frame 3, 92 {
              }
              frame 2, 76 {
              }
            }
            n165 = Get Date/Time In Seconds() -> (seconds since 1Jan1904=w348:timestamp)
            n166 = Bundle By Name(cluster=T16 {"时间标识"=timestamp(0 s since 1904-01-01), "设备"="", "日志信息"=""} ("data in"), "时间标识"=w348, "设备"=w347, "日志信息"=w345) -> (w349:T16)
            n167 = call "总磷总氮报警信息.vi"("data in"=w349) -> ()  [unwired: 10 in, 1 out]
          }
        }
      }
    }
    n168 = case shown="真" w198 {
      frame False {
      }
      frame True {
        n169 = property on="多列列表框" class="MCListbox (严格)"() -> ("ItemNames"=w278:string[][], "Value"=w279:i32)  [unwired: 2 in, 2 out]
        n170 = Index Array(array=w278, index (row)=w279) -> (element=w277:string[])  [unwired: 1 in]
        n171 = Index Array(array=w277) -> (element=w276:string)  [unwired: 1 in]
        n172 = case shown="\"初始化\", \"读空白\", \"读取比色值\", \"读取空白值\", \"读数\", \"关闭电磁阀\", \"关阀\", \"加热消解\", \"降温\", \"结束\", \"进水样\", \"清洗\", \"清洗1\", \"润洗\", \"显色\", \"消解\", \"注入水样\"" w276 {
          selector: w276 -> [_ w282]
          frame Default {
          }
          frame "初始化", "读空白", "读取比色值", "读取空白值", "读数", "关闭电磁阀", "关阀", "加热消解", "降温", "结束", "进水样", "清洗", "清洗1", "润洗", "显色", "消解", "注入水样" {
            n173 = case shown="\"读数\"" w282 {
              selector: w282 -> [w286 w288]
              tunnel: [w286 w288] -> w281
              tunnel: [string[] [] ("数组") "数组"] -> w280
              frame "读数" {
              }
              frame Default {
              }
            }
            n174 = for {
              N: 1 -> [_]
              tunnel: w281 -> [w290]
              shift-right: [w289] -> w283
              shift-left: w280 -> [w291]
              n175 = Search 1D Array(1D array=w291, element=w290) -> (index of element=w294:i32)  [unwired: 1 in]
              n176 = Format Into String(format string="%s" ("格式字符串"), w290) -> (resulting string=w295:string)  [unwired: 2 in, 1 out]
              n177 = Equal?(x=w294, y=-1) -> (x = y?=w292:bool)
              n178 = case shown="真" w292 {
                tunnel: w295 -> [_ w303]
                tunnel: w291 -> [w297 w307]
                tunnel: w290 -> [_ w306]
                tunnel: [w297 w305] -> w289
                frame False {
                }
                frame True {
                  n179 = Insert Into Array(array=w307, new element=w306) -> (w305:string[])  [unwired: 1 in]
                  n180 = case shown="\"结束\"" w303 {
                    selector: w303 -> [w332 w335 w338]
                    tunnel: [w332 w334 w337] -> w302
                    frame Default {
                    }
                    frame "初始化" {
                      n181 = Concatenate Strings("-->>" ("字符串"), w335) -> (w334:string)
                    }
                    frame "结束" {
                      n182 = Concatenate Strings("-->>" ("字符串"), w338) -> (w337:string)
                    }
                  }
                  n183 = global read "VAR总磷总氮全局变量.vi" "状态告警区"() -> (w301:T4)
                  n184 = Unbundle By Name(w301) -> ("工作状态"=w300:T12)
                  n185 = global read "VAR总磷总氮全局变量.vi" "状态告警区"() -> (w322:T4)
                  n186 = case shown="\"水样测试\"" w300 {
                    tunnel: [_ "【水样测试】" ("字符串") "【标样核查】" ("字符串") "【零点核查】" ("字符串") "【跨度核查】" ("字符串") "【空白测试】" ("字符串") "【平行样测试】" ("字符串") "【加标回收】" ("字符串") "【空白校准】" ("字符串") "【标样校准】" ("字符串")] -> w298
                    frame "空闲", Default {
                    }
                    frame "水样测试" {
                    }
                    frame "标样核查" {
                    }
                    frame "零点核查" {
                    }
                    frame "跨度核查" {
                    }
                    frame "空白测试" {
                    }
                    frame "平行样测试" {
                    }
                    frame "加标回收" {
                    }
                    frame "空白校准" {
                    }
                    frame "标样校准" {
                    }
                  }
                  n187 = Unbundle By Name(w322) -> ("id"=w321:u16)
                  n188 = global read "VAR总磷总氮全局变量.vi" "状态告警区"() -> (w317:T4)
                  n189 = case shown="3, 92" w321 {
                    tunnel: [_ "总磷" ("table输入") "氨氮" ("table输入") "总氮" ("table输入")] -> w319
                    frame Default {
                    }
                    frame 1, 131 {
                    }
                    frame 3, 92 {
                    }
                    frame 2, 76 {
                    }
                  }
                  n190 = Unbundle By Name(w317) -> ("F0"=w314:sgl, "F1"=w313:sgl, "F2"=w312:sgl, "F3"=w311:sgl, "id"=w310:u16, "flowid"=w309:u16, "量程"=w308:u16)
                  n191 = Concatenate Strings(w298, w302) -> (w299:string)
                  n192 = Format Into String(format string="F0=%#f,F1=%#f,F2=%#f,F3=%#f,Flow=%d-%-d-%-d" ("格式字符串"), w314, w313, w312, w311, w310, w309, w308) -> (resulting string=w315:string)  [unwired: 2 in, 1 out]
                  n193 = Get Date/Time In Seconds() -> (seconds since 1Jan1904=w318:timestamp)
                  n194 = Bundle By Name(cluster=T15 {"时间标识"=timestamp(0 s since 1904-01-01), "设备"="", "日志信息"="", "流程参数"=""} ("data in"), "时间标识"=w318, "设备"=w319, "日志信息"=w299, "流程参数"=w315) -> (w320:T15)
                  n195 = call "总磷总氮操作日志.vi"("data in"=w320) -> ()  [unwired: 11 in]
                }
              }
            }
            n196 = local write "数组"(w283) -> ()
          }
        }
      }
    }
    n197 = call <vilib>:"Boolean Crossing PtByPt.vi"("input"=w225) -> ("crossing"=w189:bool)  [unwired: 2 in]
    n198 = Bundle By Name(cluster=T14 {"启动模式"=enum."跨度核查", "启动参数"=1, "量程"=enum."低量程"} ("参数簇"), "启动参数"=w220, "启动模式"=w222, "量程"=w221) -> (w214:T14)
    n199 = First Call?() -> (First Call?: T/F=w226:bool)
    n200 = Or(x=w189, y=w226) -> (x .or. y?=w224:bool)
    n201 = while {
      tunnel: w224 -> [w424]
      tunnel: w214 -> [w423]
      shift-right: [w418] -> _
      shift-left: _ -> [w420]
      shift-right: [w419] -> _
      shift-left: _ -> [w421]
      stop <- TRUE stop-if-true
      n202 = case shown="真" w424 {
        tunnel: [w426 w434] -> w419
        tunnel: [w425 w433] -> w418
        tunnel: w423 -> [_ w428]
        tunnel: w421 -> [w426 _]
        tunnel: w420 -> [w425 _]
        frame False {
        }
        frame True {
          n203 = call "斯坦道XML解析.vi"("添加的路径"="流程路径", "参数簇"=w428) -> ("步骤时间"=w429:string[], "步骤名"=w431:string[])  [unwired: 8 in]
          n204 = for {
            tunnel: w431 -> [_] mode=indexing
            tunnel: [w435] -> w432 mode=indexing
            i -> [w435]
          }
          n205 = Build Array(w431, w429) -> (w430:string[][])
          n206 = Transpose 2D Array(2D array=w430) -> (transposed array=w433:string[][])
          n207 = Number To Decimal String(number=w432) -> (decimal integer string=w434:string[])  [unwired: 1 in]
        }
      }
      n208 = property on="多列列表框" class="MCListbox (严格)"("ItemNames"=w418, "RowHdrs[]"=w419) -> ()  [unwired: 2 in, 2 out]
    }
    n209 = case shown="\"缺试剂告警\", 默认" w208 {
      selector: w208 -> [_ w365]
      tunnel: w211 -> [_ w366]
      tunnel: w210 -> [_ w364]
      frame "无告警" {
      }
      frame "缺试剂告警", Default {
        n210 = case shown="真" w364 {
          tunnel: w366 -> [_ w373]
          tunnel: w365 -> [_ w367]
          frame False {
          }
          frame True {
            n211 = case shown="\"无告警\"" w367 {
              selector: w367 -> [w375 _ _ _ _ _ _ _ _ _ _ _ _ _ _ _ _ _ _ _ _ _ _ _ _ _ _ _ _ _ _ _ _ _ _ _ _ _]
              tunnel: [w374 "无告警" "缺试剂告警" "缺水样告警" "缺蒸馏水告警" "缺标液告警" "仪表漏液告警" "标定异常告警" "超量程告警" "加热异常" "低试剂预警" "超上限告警" "超下限告警" "仪表内部其他异常" "滴定异常告警" "电极异常告警" "量程切换告警" "参数设置告警" "PH电极电位异常" "电导率电极异常" "浊度光度异常" "溶解氧电极异常" "溶解氧光强异常" "温度异常告警" "PH异常告警" "溶解氧异常告警" "电导率异常告警" "浊度异常告警" "叶绿素异常告警" "藻密度异常告警" "蓝绿藻异常告警" "ORP异常告警" "氨氮异常告警" "清洁刷异常告警" "SD卡异常告警" "蓝牙异常告警" "WiFi异常告警" "流程异常告警"] -> w368
              frame Default {
                n212 = Format Into String(format string="%d" ("格式字符串"), initial string="未知" ("工作状态"), w375) -> (resulting string=w374:string)  [unwired: 1 in, 1 out]
              }
              frame "无告警" {
              }
              frame "缺试剂告警" {
              }
              frame "缺水样告警" {
              }
              frame "缺蒸馏水告警" {
              }
              frame "缺标液告警" {
              }
              frame "仪表漏液告警" {
              }
              frame "标定异常告警" {
              }
              frame "超量程告警" {
              }
              frame "加热异常" {
              }
              frame "低试剂预警" {
              }
              frame "超上限告警" {
              }
              frame "超下限告警" {
              }
              frame "仪表内部其他异常" {
              }
              frame "滴定异常告警" {
              }
              frame "电极异常告警" {
              }
              frame "量程切换告警" {
              }
              frame "参数设置告警" {
              }
              frame "PH电极电位异常" {
              }
              frame "电导率电极异常" {
              }
              frame "浊度光度异常" {
              }
              frame "溶解氧电极异常" {
              }
              frame "溶解氧光强异常" {
              }
              frame "温度异常告警" {
              }
              frame "PH异常告警" {
              }
              frame "溶解氧异常告警" {
              }
              frame "电导率异常告警" {
              }
              frame "浊度异常告警" {
              }
              frame "叶绿素异常告警" {
              }
              frame "藻密度异常告警" {
              }
              frame "蓝绿藻异常告警" {
              }
              frame "ORP异常告警" {
              }
              frame "氨氮异常告警" {
              }
              frame "清洁刷异常告警" {
              }
              frame "SD卡异常告警" {
              }
              frame "蓝牙异常告警" {
              }
              frame "Wifi异常告警" {
              }
              frame "流程异常告警" {
              }
            }
            n213 = case shown="3, 92" w373 {
              tunnel: ["总磷" ("table输入") "氨氮" ("table输入") "总氮" ("table输入")] -> w369
              frame 1, 131 {
              }
              frame 3, 92 {
              }
              frame 2, 76, Default {
              }
            }
            n214 = Get Date/Time In Seconds() -> (seconds since 1Jan1904=w370:timestamp)
            n215 = Bundle By Name(cluster=T16 {"时间标识"=timestamp(0 s since 1904-01-01), "设备"="", "日志信息"=""} ("data in"), "时间标识"=w370, "设备"=w369, "日志信息"=w368) -> (w371:T16)
            n216 = call "总磷总氮报警信息.vi"("data in"=w371) -> ()  [unwired: 10 in, 1 out]
          }
        }
      }
    }
  }
  n217 = Bundle("参数下拉列表"=w2, "测量模式下拉列表"=w3, "量程下拉列表"=w1) -> (w4:T19)  [unwired: 1 in]
  n218 = property on="曲线模型" class="曲线模型 (严格)"("属性"=w4) -> (error out=w5:errorcluster)  [unwired: 2 in, 1 out]
  n219 = control-ref of="测量模式下拉列表"() -> (w13:refnum<vi>)
  n220 = control-ref of="量程切换阈值"() -> (w11:refnum<vi>)
  n221 = control-ref of="参数下拉列表"() -> (w14:refnum<vi>)
  n222 = control-ref of="量程下拉列表"() -> (w15:refnum<vi>)
  n223 = control-ref of="备用系数"() -> (w10:refnum<vi>)
  n224 = control-ref of="公式"() -> (w12:refnum<vi>)
  n225 = Obtain Queue(name (unnamed)="TP" ("名称（未命名）"), element data type=cluster{"命令":string, "data":variant} {"命令"="", "data"=variant}) -> (queue out=w17:refnum<queue>, error out=w18:errorcluster)  [unwired: 3 in, 1 out]
  n226 = while {
    tunnel: w17 -> [w454]
    tunnel: w18 -> [_]
    shift-right: [w452] -> _
    shift-left: enum16{"总磷", "总氮"}."总磷" ("枚举") -> [w453]
    stop <- FALSE stop-if-true
    n227 = Get Queue Status(queue=w454) -> (queue out=w448:refnum<queue>, # elements in queue=w447:i32)  [unwired: 2 in, 6 out]
    n228 = Wait (ms)(milliseconds to wait=u32 1000 ("等待时间（毫秒）")) -> ()  [unwired: 1 out]
    n229 = case shown="0" w447 {
      tunnel: w453 -> [w457 w477]
      tunnel: [w457 w476] -> w452
      tunnel: w448 -> [_ w475]
      frame Default {
      }
      frame 0 {
        # "试剂填充 172 \n管路清洗108\n氨氮92\n总磷131\n总磷海水147\n总氮76\n总氮海水92"
        n230 = case shown="\"总氮\", 默认" w477 {
          selector: w477 -> [w481 w483]
          tunnel: [w482 w484] -> w467
          tunnel: [w481 w483] -> w466
          frame "总氮", Default {
            w482 = u16 2 items=["总磷"=1, "总氮"=2] ("站号")
          }
          frame "总磷" {
            w484 = u16 1 items=["总磷"=1, "氨氮"=3] ("站号")
          }
        }
        n231 = global read "VAR总磷总氮全局变量.vi" "状态告警区"() -> (w458:T4)
        n232 = Unbundle By Name(w458) -> ("系统时间"=w465:timestamp)
        n233 = Get Date/Time In Seconds() -> (seconds since 1Jan1904=w464:timestamp)
        n234 = Bundle By Name(cluster=cluster{"命令":string, "data":variant} {"命令"="", "data"=variant} ("元素"), "命令"="读状态告警区", "data"=w467) -> (w473:cluster{"命令":string, "data":variant})
        n235 = Subtract(x=w464, y=w465) -> (x-y=w463:dbl)
        n236 = Bundle By Name(cluster=cluster{"命令":string, "data":variant} {"命令"="", "data"=variant} ("元素"), "命令"="读测量数据区", "data"=w467) -> (w470:cluster{"命令":string, "data":variant})
        n237 = Enqueue Element(queue=w475, element=w473) -> (queue out=w468:refnum<queue>)  [unwired: 2 in, 2 out]
        n238 = Absolute Value(x=w463) -> (abs(x)=w462:dbl)
        n239 = Enqueue Element(queue=w468, element=w470) -> (queue out=w459:refnum<queue>)  [unwired: 2 in, 2 out]
        n240 = Greater Or Equal?(x=w462, y=120.0) -> (x >= y?=w460:bool)
        n241 = case shown="真" w460 {
          tunnel: w459 -> [_ w479]
          frame False {
          }
          frame True {
            n242 = call "总磷总氮启动命令.vi"("参数"=T20 {"站号"=3, "量程切换"=enum."AUTO", "控制命令"=enum."校时", "模式设置"=enum."待机", "测量间隔"=0}) -> ("启动命令"=w478:cluster{"命令":string, "data":variant})  [unwired: 10 in]
            n243 = Enqueue Element(queue=w479, element=w478) -> ()  [unwired: 2 in, 3 out]
          }
        }
        n244 = Increment(x=w466) -> (x+1=w476:enum16{"总磷", "总氮"})
      }
    }
    n245 = global read "总磷总氮断电保存全局变量.vi" "流程路径"() -> (w451:path)
    n246 = global read "总磷总氮断电保存全局变量.vi" "VISA Resource"() -> (→"字符串 2":refnum<visa-resource-name>)
    n247 = global read "总磷总氮断电保存全局变量.vi" "总氮稀释倍数"() -> (→"总氮稀释倍数":dbl)
    n248 = local write "流程路径"(w451) -> ()
  }
  n249 = while {
    tunnel: w17 -> [w491]
    tunnel: w15 -> [w490]
    tunnel: w14 -> [w489]
    tunnel: w13 -> [w488]
    tunnel: w12 -> [w487]
    tunnel: w11 -> [w486]
    tunnel: w10 -> [w485]
    tunnel: w5 -> [_]
    stop <- FALSE stop-if-true
    n250 = event shown="[1] \"测量模式下拉列表\", \"量程下拉列表\", \"参数下拉列表\": 值改变" {
      selector: _ -> [_ _ _ _ _ _ _ _ _ _ _ _ _ _ _ _ _ _ _ _ _ _ _ _]
      dyn-events: _ -> [_ _ _ _ _ _ _ _ _ _ _ _ _ _ _ _ _ _ _ _ _ _ _ _]
      timeout: _ -> [_ _ _ _ _ _ _ _ _ _ _ _ _ _ _ _ _ _ _ _ _ _ _ _]
      tunnel: w491 -> [_ _ w507 w535 _ _ _ _ _ _ _ w622 _ w647 w651 _ _ _ _ _ _ _ _ _]
      tunnel: w490 -> [_ _ _ _ _ _ _ _ _ _ _ _ _ _ _ _ _ _ w667 _ w687 w696 _ _]
      tunnel: w489 -> [_ _ _ _ _ _ _ _ _ _ _ _ _ _ _ _ _ _ w665 _ w685 w698 w706 w713]
      tunnel: w488 -> [_ _ _ _ _ _ _ _ _ _ _ _ _ _ _ _ _ _ w666 _ w686 w697 _ _]
      tunnel: w487 -> [_ _ _ _ _ _ _ _ _ _ _ _ _ _ _ _ _ _ w661 _ _ _ _ _]
      tunnel: w486 -> [_ _ _ _ _ _ _ _ _ _ _ _ _ _ _ _ _ _ _ _ w681 _ _ _]
      tunnel: w485 -> [_ _ _ _ _ _ _ _ _ _ _ _ _ _ _ _ _ _ _ _ _ _ w704 _]
      tunnel: [_ w493 _ _ _ _ _ _ _ _ _ _ _ _ _ _ _ _ _ _ _ _ _ _] -> _
      event Timeout {
        n251 = event-data() -> ()  [unwired: 1 in, 3 out]
      }
      event "测量模式下拉列表", "量程下拉列表", "参数下拉列表": Value Change {
        n252 = event-data() -> ()  [unwired: 1 in, 6 out]
        n253 = local read "测量模式下拉列表"() -> (w495:enum16{"水样测量", "零点核查", "跨度核查", "标样核查", "加标回收"})
        n254 = local read "参数下拉列表"() -> (w496:enum16{"总磷", "总氮"})
        n255 = local read "量程下拉列表"() -> (w497:enum16{"低量程", "高量程"})
        n256 = Bundle("参数下拉列表"=w496, "测量模式下拉列表"=w495, "量程下拉列表"=w497) -> (w494:T19)  [unwired: 1 in]
        n257 = property on="曲线模型" class="曲线模型 (严格)"("属性"=w494) -> (error out=w493:errorcluster)  [unwired: 2 in, 1 out]
      }
      event "串口设置": Value Change {
        n258 = event-data() -> ()  [unwired: 1 in, 6 out]
        n259 = global read "总磷总氮断电保存全局变量.vi" "MB通信方式选择"() -> (w498:enum16{"串口", "TCP"})
        n260 = global read "总磷总氮断电保存全局变量.vi" "VISA Resource"() -> (w504:refnum<visa-resource-name>)
        n261 = global read "总磷总氮断电保存全局变量.vi" "PORT"() -> (w502:string)
        n262 = global read "总磷总氮断电保存全局变量.vi" "IP"() -> (w503:string)
        n263 = call "串口配置.vi"("PORT"=w502, "IP"=w503, "MB通信方式选择"=w498, "请选择串口:"=w504) -> ("PORT 2"=w500:string, "IP 2"=w501:string, "确认 2"=w505:bool, "VISA资源名称 2"=w506:refnum<visa-resource-name>, "MB通信方式选择 2"=w499:enum16{"串口", "TCP"})  [unwired: 3 in]
        n264 = case shown="真" w505 {
          tunnel: w506 -> [_ w512]
          tunnel: w507 -> [_ w511]
          tunnel: w501 -> [_ w510]
          tunnel: w500 -> [_ w509]
          tunnel: w499 -> [_ w508]
          frame False {
          }
          frame True {
            n265 = flat-sequence {
              tunnel: w512 -> [w517]
              tunnel: w511 -> [w518]
              tunnel: w510 -> [w516]
              tunnel: w509 -> [w515]
              tunnel: w508 -> [w514]
              frame #0 {
                n266 = global write "总磷总氮断电保存全局变量.vi" "IP"(w516) -> ()
                n267 = global write "总磷总氮断电保存全局变量.vi" "PORT"(w515) -> ()
                n268 = global write "总磷总氮断电保存全局变量.vi" "VISA Resource"(w517) -> ()
                n269 = global write "总磷总氮断电保存全局变量.vi" "MB通信方式选择"(w514) -> ()
                n270 = Flush Queue(queue=w518) -> (queue out=w513:refnum<queue>)  [unwired: 1 in, 2 out]
                n271 = Enqueue Element(queue=w513, element=cluster{"命令":string, "data":variant} {"命令"="启用模块", "data"=variant} ("元素")) -> ()  [unwired: 2 in, 3 out]
              }
              frame #1 {
                n272 = call <vilib>:"Application Directory.vi"() -> ("Application Directory"=w533:path)
                n273 = Build Path(base path=w533, name or relative path="data\\sys.ini" ("名称或相对路径")) -> (appended path=w531:path)
                n274 = call <vilib>:"Open Config Data.vi"("configuration file path"=w531) -> ("error out"=w527:errorcluster, "refnum"=w530:T13)  [unwired: 8 in, 1 out]
                n275 = vi-ref "斯坦道总磷总氮.lvlib:总磷总氮断电保存全局变量.vi"() -> (w529:refnum<vi>)
                n276 = call <userlib>:"Write Panel to INI__ogtk.vi"("error in (no error)"=w527, "VI ref"=w529, "refnum"=w530) -> ("error out"=w526:errorcluster, "refnum out"=w528:T13)  [unwired: 7 in]
                n277 = call <vilib>:"Close Config Data.vi"("error in (no error)"=w526, "refnum"=w528) -> ("error out"=w521:errorcluster, "file path"=w520:path)  [unwired: 8 in]
                n278 = Open/Create/Replace File(file path (use dialog)=w520, error in=w521) -> (refnum out=w524:refnum<file>, error out=w525:errorcluster)  [unwired: 4 in, 1 out]
                n279 = Flush File(refnum=w524, error in=w525) -> (refnum out=w523:refnum<file>, error out=w522:errorcluster)
                n280 = Close File(refnum=w523, error in=w522) -> ()  [unwired: 2 out]
              }
            }
          }
        }
      }
      event "模块启用": Value Change {
        n281 = event-data() -> ("OldVal"=w536:bool)  [unwired: 1 in, 5 out]
        n282 = Flush Queue(queue=w535) -> (queue out=w534:refnum<queue>)  [unwired: 1 in, 2 out]
        n283 = case shown="假" w536 {
          tunnel: w534 -> [w537 w539]
          frame False {
            n284 = Enqueue Element(queue=w537, element=cluster{"命令":string, "data":variant} {"命令"="停用模块", "data"=variant} ("元素")) -> ()  [unwired: 2 in, 3 out]
          }
          frame True {
            n285 = Enqueue Element(queue=w539, element=cluster{"命令":string, "data":variant} {"命令"="启用模块", "data"=variant} ("元素")) -> ()  [unwired: 2 in, 3 out]
          }
        }
      }
      event "总氮稀释倍数": Value Change {
        n286 = event-data() -> ()  [unwired: 1 in, 6 out]
        n287 = flat-sequence {
          frame #0 {
            n288 = local read "总氮稀释倍数"() -> (w541:dbl)
            n289 = global write "总磷总氮断电保存全局变量.vi" "总氮稀释倍数"(w541) -> ()
          }
          frame #1 {
            n290 = call <vilib>:"Application Directory.vi"() -> ("Application Directory"=w555:path)
            n291 = Build Path(base path=w555, name or relative path="data\\sys.ini" ("名称或相对路径")) -> (appended path=w553:path)
            n292 = call <vilib>:"Open Config Data.vi"("configuration file path"=w553) -> ("error out"=w549:errorcluster, "refnum"=w552:T13)  [unwired: 8 in, 1 out]
            n293 = vi-ref "总磷总氮断电保存全局变量.vi"() -> (w551:refnum<vi>)
            n294 = call <userlib>:"Write Panel to INI__ogtk.vi"("error in (no error)"=w549, "VI ref"=w551, "refnum"=w552) -> ("error out"=w548:errorcluster, "refnum out"=w550:T13)  [unwired: 7 in]
            n295 = call <vilib>:"Close Config Data.vi"("error in (no error)"=w548, "refnum"=w550) -> ("error out"=w543:errorcluster, "file path"=w542:path)  [unwired: 8 in]
            n296 = Open/Create/Replace File(file path (use dialog)=w542, error in=w543) -> (refnum out=w546:refnum<file>, error out=w547:errorcluster)  [unwired: 4 in, 1 out]
            n297 = Flush File(refnum=w546, error in=w547) -> (refnum out=w545:refnum<file>, error out=w544:errorcluster)
            n298 = Close File(refnum=w545, error in=w544) -> ()  [unwired: 2 out]
          }
        }
      }
      event "流程路径": Value Change {
        n299 = event-data() -> ()  [unwired: 1 in, 6 out]
        n300 = flat-sequence {
          frame #0 {
            n301 = local read "流程路径"() -> (w556:path)
            n302 = global write "总磷总氮断电保存全局变量.vi" "流程路径"(w556) -> ()
          }
          frame #1 {
            n303 = call <vilib>:"Application Directory.vi"() -> ("Application Directory"=w570:path)
            n304 = Build Path(base path=w570, name or relative path="data\\sys.ini" ("名称或相对路径")) -> (appended path=w568:path)
            n305 = call <vilib>:"Open Config Data.vi"("configuration file path"=w568) -> ("error out"=w564:errorcluster, "refnum"=w567:T13)  [unwired: 8 in, 1 out]
            n306 = vi-ref "总磷总氮断电保存全局变量.vi"() -> (w566:refnum<vi>)
            n307 = call <userlib>:"Write Panel to INI__ogtk.vi"("error in (no error)"=w564, "VI ref"=w566, "refnum"=w567) -> ("error out"=w563:errorcluster, "refnum out"=w565:T13)  [unwired: 7 in]
            n308 = call <vilib>:"Close Config Data.vi"("error in (no error)"=w563, "refnum"=w565) -> ("error out"=w558:errorcluster, "file path"=w557:path)  [unwired: 8 in]
            n309 = Open/Create/Replace File(file path (use dialog)=w557, error in=w558) -> (refnum out=w561:refnum<file>, error out=w562:errorcluster)  [unwired: 4 in, 1 out]
            n310 = Flush File(refnum=w561, error in=w562) -> (refnum out=w560:refnum<file>, error out=w559:errorcluster)
            n311 = Close File(refnum=w560, error in=w559) -> ()  [unwired: 2 out]
          }
        }
      }
      event "公式一键写入": Value Change {
        n312 = event-data() -> ()  [unwired: 1 in, 6 out]
        n313 = local read "公式"() -> (w571:cluster{"X^2":dbl, "X":dbl, "b":dbl})
        n314 = call "公式复合写入.vi"("公式"=w571) -> ()  [unwired: 11 in]
      }
      event "备用系数一键写入": Value Change {
        n315 = event-data() -> ()  [unwired: 1 in, 6 out]
        n316 = local read "备用系数"() -> (w572:T2)
        n317 = call "量程参数复合参数写入.vi"("备用系数"=w572) -> ()  [unwired: 11 in]
      }
      event "曲线模型": Value Change {
        n318 = event-data() -> ()  [unwired: 1 in, 6 out]
        n319 = local write "公式"("曲线模型") -> ()
      }
      event "质控参数设置": Value Change {
        n320 = event-data() -> ()  [unwired: 1 in, 6 out]
        n321 = global read "总磷总氮断电保存全局变量.vi" "质控参数设置"() -> (w574:T21)
        n322 = call "总磷总氮质控参数设置.vi"("质控参数设置"=w574) -> ("输出簇"=w575:T22)  [unwired: 10 in]
        n323 = Unbundle By Name(w575) -> ("确定"=w576:bool)
        n324 = case shown="真" w576 {
          tunnel: w575 -> [_ w578]
          tunnel: w574 -> [_ w577]
          frame False {
          }
          frame True {
            n325 = flat-sequence {
              tunnel: w578 -> [w589]
              tunnel: w577 -> [w588]
              frame #0 {
                n326 = Unbundle By Name(w589) -> ("总磷跨度值"=w587:dbl, "总磷零点标准液浓度"=w586:dbl, "总磷跨度标准液浓度"=w585:dbl, "总磷标准液标准浓度"=w584:dbl, "总氮跨度值"=w583:dbl, "总氮零点标准液浓度"=w582:dbl, "总氮跨度标准液浓度"=w581:dbl, "总氮标准液标准浓度"=w580:dbl)
                n327 = Bundle By Name(cluster=w588, "总磷跨度值"=w587, "总磷零点标准液浓度"=w586, "总磷跨度标准液浓度"=w585, "总磷标准液标准浓度"=w584, "总氮跨度值"=w583, "总氮零点标准液浓度"=w582, "总氮跨度标准液浓度"=w581, "总氮标准液标准浓度"=w580) -> (w579:T21)
                n328 = global write "总磷总氮断电保存全局变量.vi" "质控参数设置"(w579) -> ()
              }
              frame #1 {
                n329 = call <vilib>:"Application Directory.vi"() -> ("Application Directory"=w603:path)
                n330 = Build Path(base path=w603, name or relative path="data\\sys.ini" ("名称或相对路径")) -> (appended path=w601:path)
                n331 = call <vilib>:"Open Config Data.vi"("configuration file path"=w601) -> ("error out"=w597:errorcluster, "refnum"=w600:T13)  [unwired: 8 in, 1 out]
                n332 = vi-ref "总磷总氮断电保存全局变量.vi"() -> (w599:refnum<vi>)
                n333 = call <userlib>:"Write Panel to INI__ogtk.vi"("error in (no error)"=w597, "VI ref"=w599, "refnum"=w600) -> ("error out"=w596:errorcluster, "refnum out"=w598:T13)  [unwired: 7 in]
                n334 = call <vilib>:"Close Config Data.vi"("error in (no error)"=w596, "refnum"=w598) -> ("error out"=w591:errorcluster, "file path"=w590:path)  [unwired: 8 in]
                n335 = Open/Create/Replace File(file path (use dialog)=w590, error in=w591) -> (refnum out=w594:refnum<file>, error out=w595:errorcluster)  [unwired: 4 in, 1 out]
                n336 = Flush File(refnum=w594, error in=w595) -> (refnum out=w593:refnum<file>, error out=w592:errorcluster)
                n337 = Close File(refnum=w593, error in=w592) -> ()  [unwired: 2 out]
              }
            }
          }
        }
      }
      event "总磷自动测试量程配置", "总氮自动测试量程配置": Value Change {
        n338 = event-data() -> ()  [unwired: 1 in, 6 out]
        n339 = flat-sequence {
          frame #0 {
            n340 = global write "总磷总氮断电保存全局变量.vi" "总氮自动测试量程配置"("总氮自动测试量程配置") -> ()
            n341 = global write "总磷总氮断电保存全局变量.vi" "总磷自动测试量程配置"("总磷自动测试量程配置") -> ()
          }
          frame #1 {
            n342 = call <vilib>:"Application Directory.vi"() -> ("Application Directory"=w619:path)
            n343 = Build Path(base path=w619, name or relative path="data\\sys.ini" ("名称或相对路径")) -> (appended path=w617:path)
            n344 = call <vilib>:"Open Config Data.vi"("configuration file path"=w617) -> ("error out"=w613:errorcluster, "refnum"=w616:T13)  [unwired: 8 in, 1 out]
            n345 = vi-ref "总磷总氮断电保存全局变量.vi"() -> (w615:refnum<vi>)
            n346 = call <userlib>:"Write Panel to INI__ogtk.vi"("error in (no error)"=w613, "VI ref"=w615, "refnum"=w616) -> ("error out"=w612:errorcluster, "refnum out"=w614:T13)  [unwired: 7 in]
            n347 = call <vilib>:"Close Config Data.vi"("error in (no error)"=w612, "refnum"=w614) -> ("error out"=w607:errorcluster, "file path"=w606:path)  [unwired: 8 in]
            n348 = Open/Create/Replace File(file path (use dialog)=w606, error in=w607) -> (refnum out=w610:refnum<file>, error out=w611:errorcluster)  [unwired: 4 in, 1 out]
            n349 = Flush File(refnum=w610, error in=w611) -> (refnum out=w609:refnum<file>, error out=w608:errorcluster)
            n350 = Close File(refnum=w609, error in=w608) -> ()  [unwired: 2 out]
          }
        }
      }
      event "手动启动": Value Change {
        n351 = event-data() -> ()  [unwired: 1 in, 6 out]
        n352 = call "总磷总氮启动参数对话框.vi"() -> ("确认"=w620:bool, "元素"=w621:cluster{"命令":string, "data":variant})  [unwired: 10 in]
        n353 = case shown="真" w620 {
          tunnel: w622 -> [_ w624]
          tunnel: w621 -> [_ w623]
          frame False {
          }
          frame True {
            n354 = Enqueue Element(queue=w624, element=w623) -> ()  [unwired: 2 in, 3 out]
          }
        }
      }
      event "定时启动": Mouse Down {
        n355 = event-data() -> ()  [unwired: 1 in, 6 out]
        n356 = flat-sequence {
          frame #0 {
            n357 = global read "总磷总氮断电保存全局变量.vi" "定时控制"() -> (w626:T6)
            n358 = call "总磷总氮周期设置.vi"("定时控制输入"=w626) -> ("定时控制输出"=w625:T23)  [unwired: 10 in]
            n359 = global write "总磷总氮断电保存全局变量.vi" "定时控制"(w625) -> ()
          }
          frame #1 {
            n360 = call <vilib>:"Application Directory.vi"() -> ("Application Directory"=w640:path)
            n361 = Build Path(base path=w640, name or relative path="data\\sys.ini" ("名称或相对路径")) -> (appended path=w638:path)
            n362 = call <vilib>:"Open Config Data.vi"("configuration file path"=w638) -> ("error out"=w634:errorcluster, "refnum"=w637:T13)  [unwired: 8 in, 1 out]
            n363 = vi-ref "总磷总氮断电保存全局变量.vi"() -> (w636:refnum<vi>)
            n364 = call <userlib>:"Write Panel to INI__ogtk.vi"("error in (no error)"=w634, "VI ref"=w636, "refnum"=w637) -> ("error out"=w633:errorcluster, "refnum out"=w635:T13)  [unwired: 7 in]
            n365 = call <vilib>:"Close Config Data.vi"("error in (no error)"=w633, "refnum"=w635) -> ("error out"=w628:errorcluster, "file path"=w627:path)  [unwired: 8 in]
            n366 = Open/Create/Replace File(file path (use dialog)=w627, error in=w628) -> (refnum out=w631:refnum<file>, error out=w632:errorcluster)  [unwired: 4 in, 1 out]
            n367 = Flush File(refnum=w631, error in=w632) -> (refnum out=w630:refnum<file>, error out=w629:errorcluster)
            n368 = Close File(refnum=w630, error in=w629) -> ()  [unwired: 2 out]
          }
        }
      }
      event "单步测试": Value Change {
        w642 = u16 1 items=["总磷"=1, "氨氮"=3] ("站号")
        n369 = event-data() -> ()  [unwired: 1 in, 6 out]
        n370 = Bundle("站号"=w642, "总磷氨氮调试"="总磷氨氮调试") -> (w641:cluster{"站号":u16, "总磷氨氮调试":u16[]})  [unwired: 1 in]
        n371 = Bundle By Name(cluster=cluster{"命令":string, "data":variant} {"命令"="", "data"=variant} ("元素"), "命令"="debug", "data"=w641) -> (w644:cluster{"命令":string, "data":variant})
        n372 = Enqueue Element(queue=w647, element=w644) -> ()  [unwired: 2 in, 3 out]
      }
      event "停止": Value Change {
        n373 = event-data() -> ()  [unwired: 1 in, 6 out]
        n374 = Enqueue Element(queue=w651, element=cluster{"命令":string, "data":variant} {"命令"="启动", "data"=variant(cluster{"站号":u16, "控制命令输出":u16[]} {"站号"=1, "控制命令输出"=[2816]})} ("元素")) -> (queue out=w648:refnum<queue>)  [unwired: 2 in, 2 out]
        n375 = Enqueue Element(queue=w648, element=cluster{"命令":string, "data":variant} {"命令"="启动", "data"=variant(cluster{"站号":u16, "控制命令输出":u16[]} {"站号"=2, "控制命令输出"=[2816]})} ("元素")) -> ()  [unwired: 2 in, 3 out]
      }
      event "设置": Value Change {
        n376 = event-data() -> ()  [unwired: 1 in, 6 out]
        n377 = property on="窗格" class="Pane"("Origin"=T10 {"Horizontal"=0, "Vertical"=628} ("原点")) -> ()  [unwired: 2 in, 2 out]
      }
      event "返回": Value Change {
        n378 = event-data() -> ()  [unwired: 1 in, 6 out]
        n379 = property on="窗格" class="Pane"("Origin"=T10 {"Horizontal"=0, "Vertical"=0} ("原点")) -> ()  [unwired: 2 in, 2 out]
      }
      event "公式.X^2", "公式.X", "公式.b", "量程切换阈值.阈值", "量程切换阈值.标液浓度", "备用系数.量程上限", "备用系数.量程下限", "备用系数.检出限", "备用系数.精度", "总氮稀释倍数": Mouse Down {
        n380 = event-data() -> ("CtlRef"=w657:refnum<vi>)  [unwired: 1 in, 5 out]
        n381 = property class="DigNum (严格)"(reference=w657) -> (reference out=w655:refnum<vi>, "Value"=w656:dbl)  [unwired: 1 in, 1 out]
        n382 = call "数字键盘.vi"("OldNumber"=w656) -> ("NewNumber"=w654:dbl)
        n383 = property class="DigNum (严格)"(reference=w655, "Val(Sgnl)"=w654) -> ()  [unwired: 1 in, 2 out]
      }
      event "读公式": Value Change {
        n384 = event-data() -> ()  [unwired: 1 in, 6 out]
        n385 = property class="Enum (严格)"(reference=w665) -> ("Value"=w664:enum16{"总磷", "总氮"})  [unwired: 1 in, 2 out]
        n386 = property class="Enum (严格)"(reference=w666) -> ("Value"=w663:enum16{"水样测量", "零点核查", "跨度核查", "标样核查", "加标回收"})  [unwired: 1 in, 2 out]
        n387 = property class="Enum (严格)"(reference=w667) -> ("Value"=w662:enum16{"低量程", "高量程"})  [unwired: 1 in, 2 out]
        n388 = call "总磷总氮公式读取.vi"("量程"=w662, "测量模式"=w663, "测量参数"=w664) -> ("error out"=w659:errorcluster, "公式"=w660:cluster{"X^2":dbl, "X":dbl, "b":dbl})  [unwired: 7 in]
        n389 = property class="Clust (严格)"(reference=w661, "Value"=w660) -> ()  [unwired: 1 in, 2 out]
        n390 = case shown="错误" w659 {
          tunnel: ["读取成功" ("消息") "读取失败" ("消息")] -> w658
          frame No Error {
          }
          frame Error {
          }
        }
        n391 = One Button Dialog(message=w658) -> ()  [unwired: 1 in, 1 out]
      }
      event "写公式": Value Change {
        n392 = event-data() -> ()  [unwired: 1 in, 6 out]
        n393 = call "总磷总氮公式写入.vi"("公式"="公式", "量程"="量程下拉列表", "测量模式"="测量模式下拉列表", "测量参数"="参数下拉列表") -> ("error out"=w672:errorcluster)  [unwired: 7 in]
        n394 = case shown="无错误" w672 {
          tunnel: ["写入成功" ("消息") "写入失败" ("消息")] -> w673
          frame No Error {
          }
          frame Error {
          }
        }
        n395 = One Button Dialog(message=w673) -> ()  [unwired: 1 in, 1 out]
      }
      event "量程切换阈值读取": Value Change {
        n396 = event-data() -> ()  [unwired: 1 in, 6 out]
        n397 = property class="Enum (严格)"(reference=w685) -> ("Value"=w684:enum16{"总磷", "总氮"})  [unwired: 1 in, 2 out]
        n398 = property class="Enum (严格)"(reference=w686) -> ("Value"=w683:enum16{"水样测量", "零点核查", "跨度核查", "标样核查", "加标回收"})  [unwired: 1 in, 2 out]
        n399 = property class="Enum (严格)"(reference=w687) -> ("Value"=w682:enum16{"低量程", "高量程"})  [unwired: 1 in, 2 out]
        n400 = call "总磷总氮量程读取.vi"("量程"=w682, "测量模式"=w683, "测量参数"=w684) -> ("error out"=w678:errorcluster, "量程切换阈值"=w680:cluster{"阈值":dbl, "标液浓度":dbl})  [unwired: 7 in]
        n401 = property class="Clust (严格)"(reference=w681, "Value"=w680) -> ()  [unwired: 1 in, 2 out]
        n402 = case shown="错误" w678 {
          tunnel: ["读取成功" ("消息") "读取失败" ("消息")] -> w679
          frame No Error {
          }
          frame Error {
          }
        }
        n403 = One Button Dialog(message=w679) -> ()  [unwired: 1 in, 1 out]
      }
      event "量程切换阈值写入": Value Change {
        n404 = event-data() -> ()  [unwired: 1 in, 6 out]
        n405 = property class="Enum (严格)"(reference=w698) -> ("Value"=w695:enum16{"总磷", "总氮"})  [unwired: 1 in, 2 out]
        n406 = property class="Enum (严格)"(reference=w697) -> ("Value"=w694:enum16{"水样测量", "零点核查", "跨度核查", "标样核查", "加标回收"})  [unwired: 1 in, 2 out]
        n407 = property class="Enum (严格)"(reference=w696) -> ("Value"=w693:enum16{"低量程", "高量程"})  [unwired: 1 in, 2 out]
        n408 = call "总磷总氮量程写入.vi"("量程切换阈值"="量程切换阈值", "量程"=w693, "测量模式"=w694, "测量参数"=w695) -> ("error out"=w690:errorcluster)  [unwired: 7 in]
        n409 = case shown="无错误" w690 {
          tunnel: ["写入成功" ("消息") "写入失败" ("消息")] -> w691
          frame No Error {
          }
          frame Error {
          }
        }
        n410 = One Button Dialog(message=w691) -> ()  [unwired: 1 in, 1 out]
      }
      event "备用系数读取": Value Change {
        n411 = event-data() -> ()  [unwired: 1 in, 6 out]
        n412 = property class="Enum (严格)"(reference=w706) -> ("Value"=w705:enum16{"总磷", "总氮"})  [unwired: 1 in, 2 out]
        n413 = call "总磷总氮备用系数读取.vi"("测量参数"=w705) -> ("error out"=w701:errorcluster, "备用系数"=w703:T2)  [unwired: 9 in]
        n414 = property class="Clust (严格)"(reference=w704, "Value"=w703) -> ()  [unwired: 1 in, 2 out]
        n415 = case shown="错误" w701 {
          tunnel: ["读取成功" ("消息") "读取失败" ("消息")] -> w702
          frame No Error {
          }
          frame Error {
          }
        }
        n416 = One Button Dialog(message=w702) -> ()  [unwired: 1 in, 1 out]
      }
      event "备用系数写入": Value Change {
        n417 = event-data() -> ()  [unwired: 1 in, 6 out]
        n418 = property class="Enum (严格)"(reference=w713) -> ("Value"=w712:enum16{"总磷", "总氮"})  [unwired: 1 in, 2 out]
        n419 = call "总磷总氮备用系数写入.vi"("备用系数"="备用系数", "测量参数"=w712) -> ("error out"=w709:errorcluster)  [unwired: 9 in]
        n420 = case shown="无错误" w709 {
          tunnel: ["写入成功" ("消息") "写入失败" ("消息")] -> w710
          frame No Error {
          }
          frame Error {
          }
        }
        n421 = One Button Dialog(message=w710) -> ()  [unwired: 1 in, 1 out]
      }
    }
  }
